vi "MojoLoader.vi"(0 "Mode":enum16{"RAM", "FLASH", "VERIFY"}(ring), 1 "Path":path, 2 "Port":refnum<visa-resource-name>) -> ()   [LabVIEW 2018]
uses:
  <vilib>/Instr/_visa.llb/VISA Configure Serial Port (Instr).vi
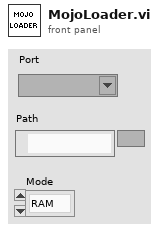
[diagram p1: front panel]
types:
  T1 = enum16{"big-endian, network order", "native, host order", "little-endian"}
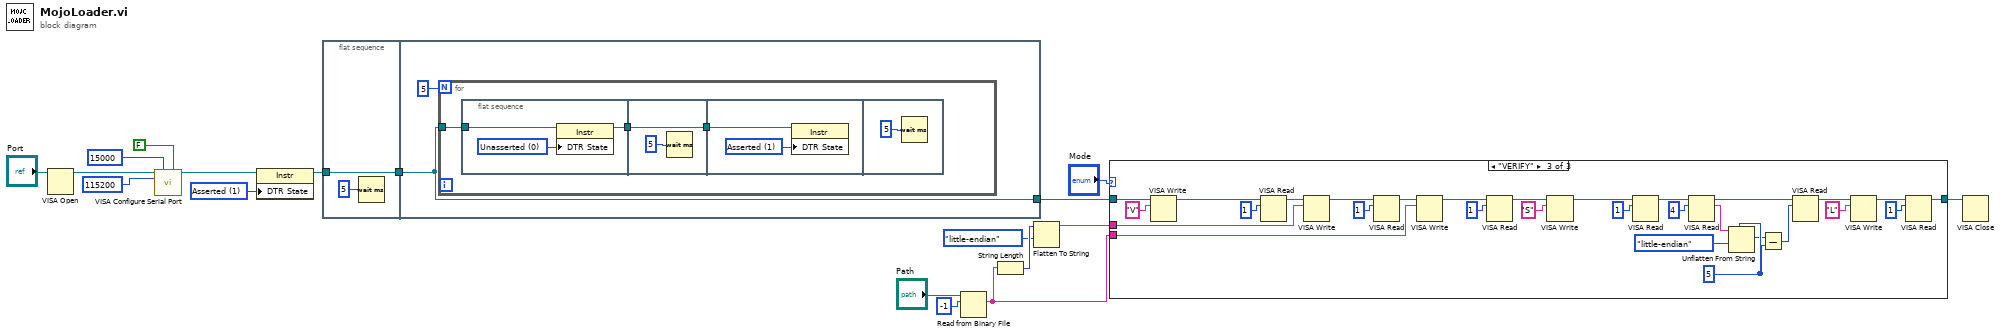
[diagram p0: block diagram]
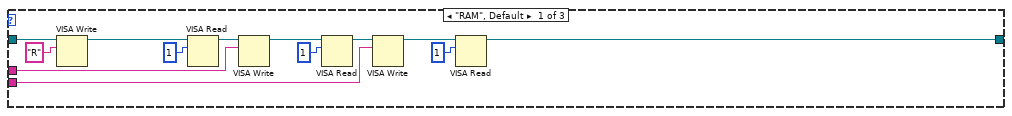
[diagram p2: hidden frame]
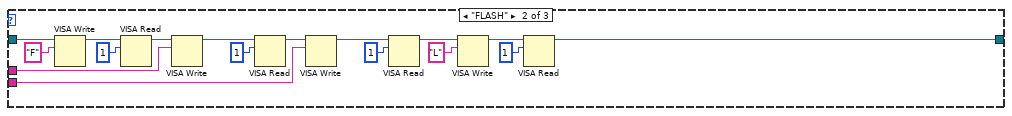
[diagram p3: hidden frame]
diagram:
  w3 = i16 1 items=["Unknown"=-1, "Unasserted"=0, "Asserted"=1] ("Serial Settings:Modem Line Settings:Line DTR State")
  n1 = VISA Open(VISA resource name="Port") -> (VISA resource name=w13:refnum<visa-resource-name>)  [unwired: 4 in, 1 out]
  n2 = call-poly "VISA Configure Serial Port"("VISA resource name"=w13, "timeout (10sec)"=u32 15000, "Enable Termination\nChar (T)"=FALSE ("Enable Termination\nChar (T)"), "baud rate (9600)"=u32 115200) -> ("VISA resource name out"=w4:refnum<visa-resource-name>)  [unwired: 10 in, 1 out]
  n3 = property class="Instr"(reference=w4, "DTR State"=w3) -> (reference out=w2:refnum<visa-resource-name>)  [unwired: 1 in, 1 out]
  n4 = flat-sequence {
    tunnel: [w19] -> w15
    tunnel: w2 -> [w19]
    tunnel: w15 -> [w21]
    tunnel: [w21] -> w5
    frame #0 {
      n5 = Wait (ms)(milliseconds to wait=u32 5) -> ()  [unwired: 1 out]
    }
    frame #1 {
      n6 = for {
        N: 5 -> [_]
        tunnel: w21 -> [w25]
        n7 = flat-sequence {
          tunnel: w25 -> [w27]
          tunnel: [w26] -> w23
          tunnel: [w29] -> w24
          tunnel: w23 -> [w29]
          tunnel: w24 -> [w31]
          frame #0 {
            w28 = i16 0 items=["Unknown"=-1, "Unasserted"=0, "Asserted"=1] ("Serial Settings:Modem Line Settings:Line DTR State")
            n8 = property class="Instr"(reference=w27, "DTR State"=w28) -> (reference out=w26:refnum<visa-resource-name>)  [unwired: 1 in, 1 out]
          }
          frame #1 {
            n9 = Wait (ms)(milliseconds to wait=u32 5) -> ()  [unwired: 1 out]
          }
          frame #2 {
            w32 = i16 1 items=["Unknown"=-1, "Unasserted"=0, "Asserted"=1] ("Serial Settings:Modem Line Settings:Line DTR State")
            n10 = property class="Instr"(reference=w31, "DTR State"=w32) -> ()  [unwired: 1 in, 2 out]
          }
          frame #3 {
            n11 = Wait (ms)(milliseconds to wait=u32 5) -> ()  [unwired: 1 out]
          }
        }
      }
    }
  }
  n12 = Read from Binary File(10:-1 ("count (1)"), 11:"Path") -> (2:w12:string)  [unwired: 4 in, 3 out]
  n13 = String Length(string=w12) -> (length=w10:i32)
  n14 = Flatten To String(anything=w10, byte order (0:big-endian, network order)=T1."little-endian") -> (data string=w11:string)  [unwired: 2 in, 2 out]
  n15 = case shown="\"VERIFY\"" "Mode" {
    tunnel: w12 -> [w45 w62 w91]
    tunnel: w11 -> [w42 w59 w88]
    tunnel: [w35 w47 w69] -> w6
    tunnel: w5 -> [w34 w52 w81]
    frame "RAM", Default {
      n16 = VISA Write(VISA resource name=w34, write buffer="R") -> (VISA resource name out=w40:refnum<visa-resource-name>)  [unwired: 1 in, 2 out]
      n17 = VISA Read(VISA resource name=w40, byte count=u32 1) -> (VISA resource name out=w41:refnum<visa-resource-name>)  [unwired: 1 in, 3 out]
      n18 = VISA Write(VISA resource name=w41, write buffer=w42) -> (VISA resource name out=w43:refnum<visa-resource-name>)  [unwired: 1 in, 2 out]
      n19 = VISA Read(VISA resource name=w43, byte count=u32 1) -> (VISA resource name out=w44:refnum<visa-resource-name>)  [unwired: 1 in, 3 out]
      n20 = VISA Write(VISA resource name=w44, write buffer=w45) -> (VISA resource name out=w46:refnum<visa-resource-name>)  [unwired: 1 in, 2 out]
      n21 = VISA Read(VISA resource name=w46, byte count=u32 1) -> (VISA resource name out=w35:refnum<visa-resource-name>)  [unwired: 1 in, 3 out]
    }
    frame "FLASH" {
      n22 = VISA Write(VISA resource name=w52, write buffer="F") -> (VISA resource name out=w57:refnum<visa-resource-name>)  [unwired: 1 in, 2 out]
      n23 = VISA Read(VISA resource name=w57, byte count=u32 1) -> (VISA resource name out=w58:refnum<visa-resource-name>)  [unwired: 1 in, 3 out]
      n24 = VISA Write(VISA resource name=w58, write buffer=w59) -> (VISA resource name out=w60:refnum<visa-resource-name>)  [unwired: 1 in, 2 out]
      n25 = VISA Read(VISA resource name=w60, byte count=u32 1) -> (VISA resource name out=w61:refnum<visa-resource-name>)  [unwired: 1 in, 3 out]
      n26 = VISA Write(VISA resource name=w61, write buffer=w62) -> (VISA resource name out=w63:refnum<visa-resource-name>)  [unwired: 1 in, 2 out]
      n27 = VISA Read(VISA resource name=w63, byte count=u32 1) -> (VISA resource name out=w48:refnum<visa-resource-name>)  [unwired: 1 in, 3 out]
      n28 = VISA Write(VISA resource name=w48, write buffer="L") -> (VISA resource name out=w49:refnum<visa-resource-name>)  [unwired: 1 in, 2 out]
      n29 = VISA Read(VISA resource name=w49, byte count=u32 1) -> (VISA resource name out=w47:refnum<visa-resource-name>)  [unwired: 1 in, 3 out]
    }
    frame "VERIFY" {
      w66 = u32 5 ("byte count")
      n30 = VISA Write(VISA resource name=w81, write buffer="V") -> (VISA resource name out=w86:refnum<visa-resource-name>)  [unwired: 1 in, 2 out]
      n31 = VISA Read(VISA resource name=w86, byte count=u32 1) -> (VISA resource name out=w87:refnum<visa-resource-name>)  [unwired: 1 in, 3 out]
      n32 = VISA Write(VISA resource name=w87, write buffer=w88) -> (VISA resource name out=w89:refnum<visa-resource-name>)  [unwired: 1 in, 2 out]
      n33 = VISA Read(VISA resource name=w89, byte count=u32 1) -> (VISA resource name out=w90:refnum<visa-resource-name>)  [unwired: 1 in, 3 out]
      n34 = VISA Write(VISA resource name=w90, write buffer=w91) -> (VISA resource name out=w92:refnum<visa-resource-name>)  [unwired: 1 in, 2 out]
      n35 = VISA Read(VISA resource name=w92, byte count=u32 1) -> (VISA resource name out=w79:refnum<visa-resource-name>)  [unwired: 1 in, 3 out]
      n36 = VISA Write(VISA resource name=w79, write buffer="S") -> (VISA resource name out=w77:refnum<visa-resource-name>)  [unwired: 1 in, 2 out]
      n37 = VISA Read(VISA resource name=w77, byte count=u32 1) -> (VISA resource name out=w75:refnum<visa-resource-name>)  [unwired: 1 in, 3 out]
      n38 = VISA Read(VISA resource name=w75, byte count=u32 4) -> (VISA resource name out=w74:refnum<visa-resource-name>, read buffer=w68:string)  [unwired: 1 in, 2 out]
      n39 = Unflatten From String(type=w66, binary string=w68, byte order (0:big-endian, network order)=T1."little-endian") -> (value=w64:u32)  [unwired: 2 in, 2 out]
      n40 = Subtract(x=w64, y=w66) -> (x-y=w65:u32)
      n41 = VISA Read(VISA resource name=w74, byte count=w65) -> (VISA resource name out=w72:refnum<visa-resource-name>)  [unwired: 1 in, 3 out]
      n42 = VISA Write(VISA resource name=w72, write buffer="L") -> (VISA resource name out=w70:refnum<visa-resource-name>)  [unwired: 1 in, 2 out]
      n43 = VISA Read(VISA resource name=w70, byte count=u32 1) -> (VISA resource name out=w69:refnum<visa-resource-name>)  [unwired: 1 in, 3 out]
    }
  }
  n44 = VISA Close(VISA resource name=w6) -> ()  [unwired: 1 in, 1 out]
